vi "NT Read and Format Entries as Tree.vi"(4 "Connected":bool, 6 "Tags to  Close":string[](array[string]), 8 "error in":errorcluster, 9 "Operation":enum16{"Update", "Clear"}(ring), 10 "Name Pattern":string, 11 "Tree Refnum":refnum<vi>) -> (0 "error out":errorcluster, 3 "Formatted Strings":cluster{"Name":string, "Value":string}[](array[cluster]))   [LabVIEW 2025]
doc: "Retrieve the entries that match the name pattern, and use the / seperators to construct the tree. Provide the reference to the tree control that you would like to be updated, or use the name/value pairs to update your own list, table, etc. Supported wildcards are * and ?."
uses:
  <vilib>/Utility/error.llb/Trim Whitespace One-Sided.vi
panel:
  in  "Tree":string(tree)
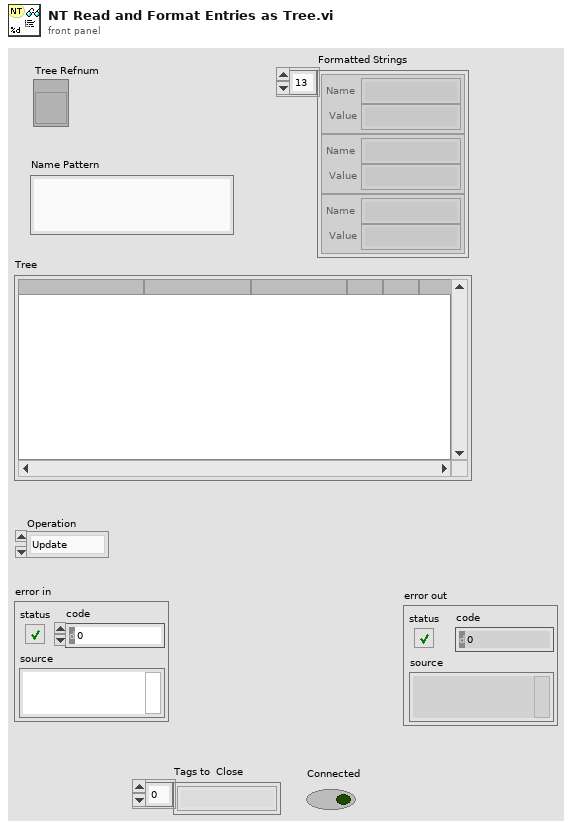
[diagram p1: front panel]
types:
  T1 = cluster{"Left Cell String":string, "Child Text":string[], "Child Tag":string, "Item Indent":i32, "Child Only?":bool, "Glyph Index":i32}[]
  T2 = cluster{"Left Cell String":string, "Child Text":string[], "Child Tag":string, "Item Indent":i32, "Child Only?":bool, "Glyph Index":i32}
  T3 = typedef "NT Datatype.ctl" = u32
  T4 = cluster{"name":string, "NT_Type":T3, "topicHandle":u32}[]
  T5 = cluster{"Array":string[], "name":string, "NT_Type":T3, "topicHandle":u32}[]
  T6 = cluster{"Left Cell String":bool, "Child Text":bool[], "Child Tag":bool, "Item Indent":bool, "Child Only?":bool, "Glyph Index":bool}[]
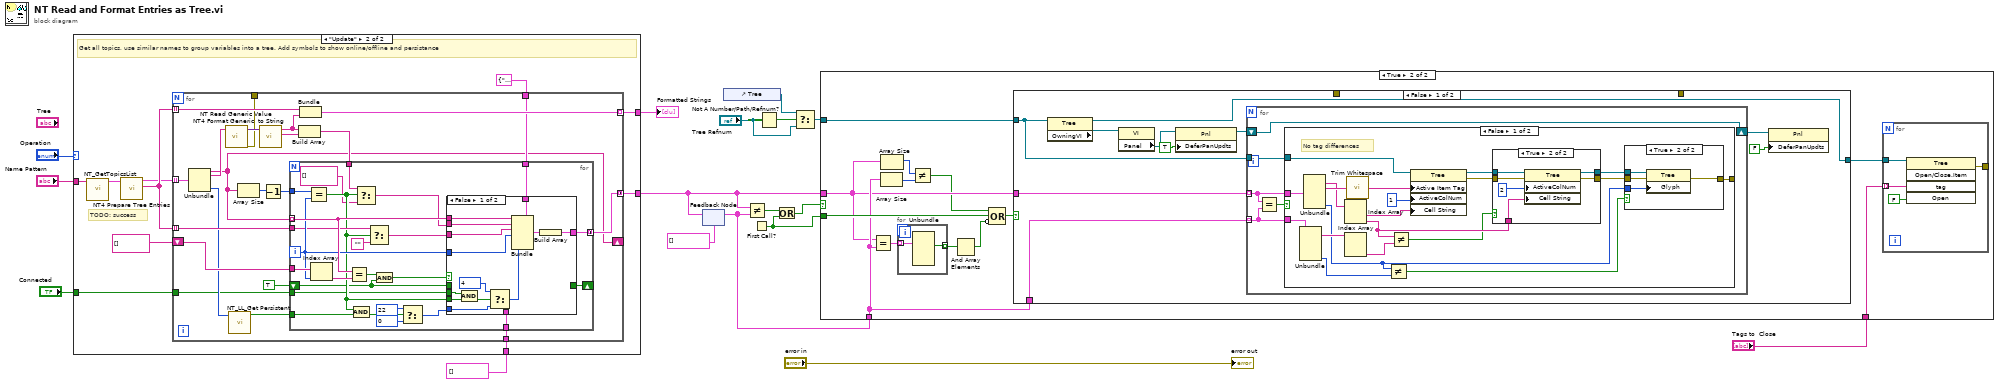
[diagram p0: block diagram]
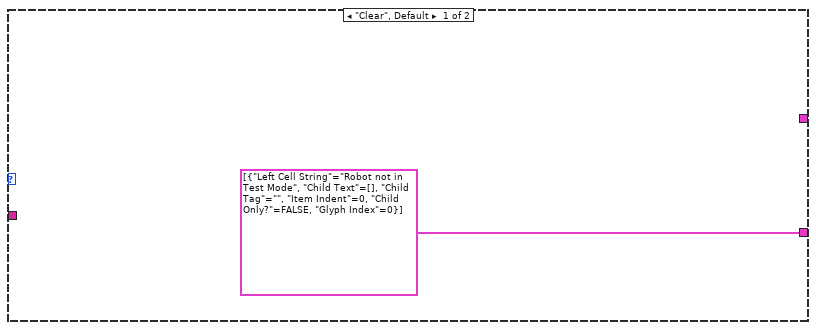
[diagram p2: hidden frame]
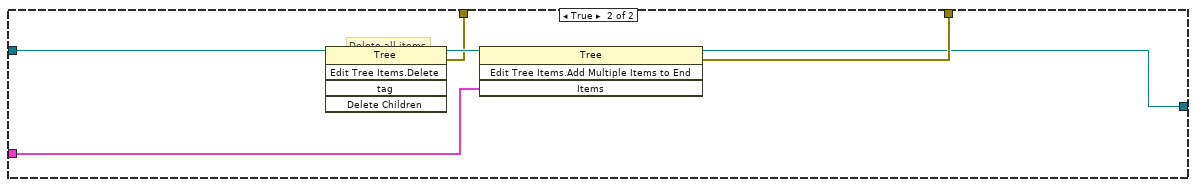
[diagram p8: hidden frame]
diagram:
  n1 = case shown="\"Update\"" "Operation" {
    tunnel: [_ w28] -> w17
    tunnel: "Name Pattern" -> [_ w23]
    tunnel: T1 [] -> [_ w26]
    tunnel: [T1 [{"Left Cell String"="Robot not in Test Mode", "Child Text"=[], "Child Tag"="", "Item Indent"=0, "Child Only?"=FALSE, "Glyph Index"=0}] w24] -> w9
    tunnel: "Connected" -> [_ w19]
    frame "Clear", Default {
    }
    frame "Update" {
      # "TODO: success"
      # "Get all topics, use similar names to group variables into a tree. Add symbols to show online/offline and persistance"
      n2 = call <vilib>:"NT_GetTopicsList.vi"("String"=w23) -> ("Topic List"=w22:T4)  [unwired: 10 in]
      n3 = call <vilib>:"NT4 Prepare Tree Entries.vi"("Topic List"=w22) -> ("Tokens"=w21:string[], "Sorted Tree Rows"=w20:T5)  [unwired: 9 in]
      n4 = for {
        tunnel: [w49] -> w28 mode=indexing
        tunnel: [w44] -> w24 mode=concatenating
        tunnel: T2 {"Left Cell String"="", "Child Text"=[], "Child Tag"="", "Item Indent"=0, "Child Only?"=FALSE, "Glyph Index"=0} ("Item") -> [w45]
        shift-right: [w30] -> _
        shift-left: string[] [] ("Child Text") -> [w47]
        tunnel: w21 -> [w48] mode=indexing
        tunnel: w26 -> [w46]
        tunnel: w21 -> [w40] mode=indexing
        tunnel: w20 -> [w38] mode=indexing
        tunnel: w19 -> [w31]
        tunnel: [w29] -> _
        n5 = Unbundle(w38) -> ("Array"=w30:string[], "name"=w37:string, "topicHandle"=w33:u32)  [unwired: 1 out]
        n6 = call <vilib>:"NT Read Generic Value.vi"("name"=w37) -> ("error out"=w29:errorcluster, "variant value"=w36:variant)  [unwired: 9 in]
        n7 = call <vilib>:"NT_LL_Get Persistent.vi"("topicHandle"=w33) -> ("Persistence"=w32:bool)  [unwired: 9 in, 1 out]
        n8 = Array Size(array=w30) -> (size(s)=w43:i32)
        n9 = call <vilib>:"NT4 Format Generic  to String.vi"("Variant"=w36) -> ("Type String"=w34:string, "String"=w35:string)  [unwired: 9 in]
        n10 = Decrement(x=w43) -> (x-1=w42:i32)
        n11 = Build Array(w35, w34) -> (w41:string[])
        n12 = for {
          tunnel: w47 -> [w74]
          tunnel: w30 -> [w69] mode=indexing
          tunnel: w46 -> [w72]
          tunnel: [w71] -> w44 mode=concatenating
          tunnel: w45 -> [w70]
          tunnel: w42 -> [w67]
          tunnel: w41 -> [w66]
          tunnel: w40 -> [w63]
          shift-right: [w59] -> _
          shift-left: TRUE -> [w51]
          tunnel: w32 -> [w53]
          tunnel: w31 -> [w52]
          i -> [w68]
          n13 = Equal?(x=w67, y=w68) -> (x = y?=w54:bool)
          n14 = Index Array(array=w74, index=w68) -> (element=w73:string)
          n15 = Equal?(x=w69, y=w73) -> (x = y?=w61:bool)
          n16 = Compound Arithmetic op=AND(w54, w53) -> (w55:bool)
          n17 = Select(t=w66, s=w54, f=string[] [] ("appended array")) -> (s? t:f=w65:string[])
          n18 = Select(t=w63, s=w54, f="") -> (s? t:f=w64:string)
          n19 = And(x=w61, y=w51) -> (x .and. y?=w60:bool)
          n20 = Select(t=22, s=w55, f=0) -> (s? t:f=w58:i32)
          n21 = case shown="False" w60 {
            tunnel: [w85 w89] -> w71
            tunnel: w72 -> [_ w89]
            tunnel: w70 -> [w87 _]
            tunnel: w69 -> [w84 _]
            tunnel: w68 -> [w83 _]
            tunnel: w65 -> [w82 _]
            tunnel: w64 -> [w81 _]
            tunnel: [_ w88] -> w59
            tunnel: w51 -> [_ w88]
            tunnel: w54 -> [w77 _]
            tunnel: w58 -> [w79 _]
            tunnel: w52 -> [w75 _]
            frame False {
              n22 = And(x=w75, y=w77) -> (x .and. y?=w76:bool)
              n23 = Select(t=4, s=w76, f=w79) -> (s? t:f=w78:i32)
              n24 = Bundle(cluster=w87, "Left Cell String"=w84, "Child Text"=w82, "Child Tag"=w81, "Item Indent"=w83, "Glyph Index"=w78) -> (w86:T2)  [unwired: 1 in]
              n25 = Build Array(w86) -> (w85:T1)
            }
            frame True {
            }
          }
        }
        n26 = Bundle(w48, "String"=w35) -> (w49:cluster{string, "String":string})  [unwired: 1 in]
      }
    }
  }
  "Formatted Strings" <- w17
  n27 = feedback #1(T1 []) -> (w3:T1)
  n28 = feedback-in #1(w9) -> ()
  n29 = control-ref of="Tree"() -> (w15:refnum<vi>)
  n30 = Not Equal?(x=w9, y=w3) -> (x != y?=w7:bool)
  n31 = First Call?() -> (First Call?: T/F=w4:bool)
  n32 = Not A Number/Path/Refnum?(number/path/refnum="Tree Refnum") -> (NaN/Path/Refnum?=w16:bool)
  n33 = Or(x=w7, y=w4) -> (x .or. y?=w8:bool)
  n34 = Select(t=w15, s=w16, f="Tree Refnum") -> (s? t:f=w5:refnum<vi>)
  n35 = case shown="True" w8 {
    tunnel: w5 -> [_ w90]
    tunnel: w9 -> [_ w96]
    tunnel: w4 -> [_ w101]
    tunnel: w3 -> [_ w97]
    tunnel: "Tags to  Close" -> [_ w92]
    frame False {
    }
    frame True {
      n36 = Equal?(x=w96, y=w97) -> (x = y?=w98:T6)
      n37 = Array Size(array=w97) -> (size(s)=w95:i32)
      n38 = Array Size(array=w96) -> (size(s)=w94:i32)
      n39 = for {
        tunnel: w98 -> [w108] mode=indexing
        tunnel: [w107] -> w102 mode=indexing
        n40 = Unbundle(w108) -> ("Child Tag"=w107:bool)  [unwired: 5 out]
      }
      n41 = Not Equal?(x=w94, y=w95) -> (x != y?=w93:bool)
      n42 = And Array Elements(Boolean array=w102) -> (logical AND=w100:bool)
      n43 = Compound Arithmetic op=OR(w93, w101, invert w100) -> (w99:bool)
      n44 = case shown="False" w99 {
        tunnel: w90 -> [w116 w161]
        tunnel: w96 -> [w118 w158]
        tunnel: w97 -> [w117 _]
        tunnel: [_ w160] -> _
        tunnel: [_ w159] -> _
        tunnel: [w109 w157] -> w91
        frame False {
          n45 = property class="Tree"(reference=w116) -> (reference out=w109:refnum<vi>, "OwningVI"=w115:refnum<vi>)  [unwired: 1 in, 1 out]
          n46 = property class="VI"(reference=w115) -> ("Panel"=w114:refnum<vi>)  [unwired: 1 in, 2 out]
          n47 = property class="Pnl"(reference=w114, "DeferPanUpdts"=TRUE) -> (reference out=w112:refnum<vi>)  [unwired: 1 in, 1 out]
          n48 = for {
            tunnel: w118 -> [w122] mode=indexing
            tunnel: w117 -> [w121] mode=indexing
            tunnel: w116 -> [w120]
            shift-right: [w119] -> w110
            shift-left: w112 -> [w119]
            n49 = Equal?(x=w122, y=w121) -> (x = y?=w123:bool)
            n50 = case shown="False" w123 {
              tunnel: w122 -> [w143 _]
              tunnel: w121 -> [w132 _]
              tunnel: w120 -> [w139 _]
              tunnel: [w134 _] -> _
              frame False {
                # "No tag differences"
                n51 = Unbundle(w132) -> ("Child Text"=w131:string[], "Glyph Index"=w126:i32)  [unwired: 4 out]
                n52 = Unbundle(w143) -> ("Child Text"=w133:string[], "Child Tag"=w142:string, "Glyph Index"=w127:i32)  [unwired: 3 out]
                n53 = Index Array(array=w133) -> (element #1=w140:string, element #2=w129:string)  [unwired: 2 in]
                n54 = Index Array(array=w131) -> (element #2=w130:string)  [unwired: 2 in, 1 out]
                n55 = call <vilib>:"Trim Whitespace.vi"("string"=w142) -> ("trimmed string"=w124:string)  [unwired: 1 in]
                n56 = Not Equal?(x=w127, y=w126) -> (x != y?=w125:bool)
                n57 = Not Equal?(x=w129, y=w130) -> (x != y?=w128:bool)
                n58 = property class="Tree"(reference=w139, "Active Item Tag"=w124, "ActiveColNum"=1 ("Active Cell:Active Column Number"), "Cell String"=w140) -> (reference out=w136:refnum<vi>, error out=w138:errorcluster)  [unwired: 1 in]
                n59 = case shown="True" w128 {
                  tunnel: w138 -> [w149 w156]
                  tunnel: [w149 w155] -> w137
                  tunnel: w136 -> [w150 w154]
                  tunnel: [w150 w153] -> w135
                  tunnel: w129 -> [_ w151]
                  frame False {
                  }
                  frame True {
                    n60 = property class="Tree"(reference=w154, error in=w156, "ActiveColNum"=2 ("Active Cell:Active Column Number"), "Cell String"=w151) -> (reference out=w153:refnum<vi>, error out=w155:errorcluster)
                  }
                }
                n61 = case shown="True" w125 {
                  tunnel: w137 -> [w144 w148]
                  tunnel: w135 -> [_ w147]
                  tunnel: [w144 w146] -> w134
                  tunnel: w127 -> [_ w145]
                  frame False {
                  }
                  frame True {
                    n62 = property class="Tree"(reference=w147, error in=w148, "Glyph"=w145) -> (error out=w146:errorcluster)  [unwired: 1 out]
                  }
                }
              }
              frame True {
              }
            }
          }
          n63 = property class="Pnl"(reference=w110, "DeferPanUpdts"=FALSE) -> ()  [unwired: 1 in, 2 out]
        }
        frame True {
          # "Delete all items"
          n64 = invoke class="Tree" method="Edit Tree Items.Delete"(reference=w161) -> (reference out=w162:refnum<vi>, error out=w160:errorcluster)  [unwired: 4 in, 3 out]
          n65 = invoke class="Tree" method="Edit Tree Items.Add Multiple Items to End"(reference=w162, "Items"=w158) -> (reference out=w157:refnum<vi>, error out=w159:errorcluster)  [unwired: 2 in, 2 out]
        }
      }
      n66 = for {
        tunnel: w92 -> [w105] mode=indexing
        tunnel: w91 -> [w106]
        tunnel: [w103] -> _
        n67 = invoke class="Tree" method="Open/Close.Item"(reference=w106, "tag"=w105, "Open"=FALSE ("Open?")) -> (error out=w103:errorcluster)  [unwired: 2 in, 4 out]
      }
    }
  }
  "error out" <- "error in"
